vi "AT+TT.vi"(8 "错误输入（无错误）":errorcluster, 11 "站号":u16) -> (0 "错误输出":errorcluster)   [LabVIEW 2016, in "斯坦道原位多参数.lvlib"]
uses:
  <vilib>/Plasmionique/MB Master/MB_Master_Serial/MB_Master_Serial.lvclass/MB_Master_Serial.ctl
  <vilib>/Plasmionique/MB Master/MB_Master_Serial/Read VISA Resource.vi
  <vilib>/Plasmionique/MB Master/MB_VISA_Lock/MB_VISA_Lock.lvlib
  <vilib>/Plasmionique/MB Master/MB_Master_Serial/MB_Master_Serial.lvclass
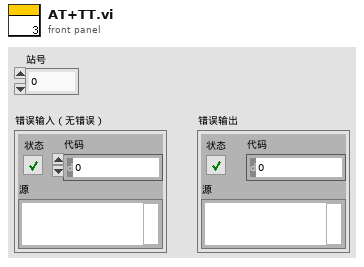
[diagram p1: front panel]
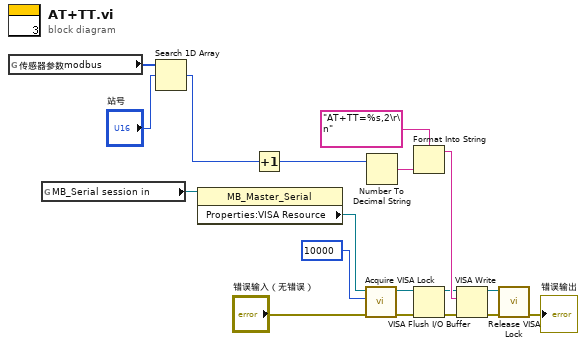
[diagram p0: block diagram]
diagram:
  n1 = global read "多参数断电保存全局变量.vi" "传感器参数modbus"() -> (w11:u16[])
  n2 = global read "多参数全局变量.vi" "MB_Serial session in"() -> (w9:refnum<class "MB_Master_Serial.lvclass">)
  n3 = Search 1D Array(1D array=w11, element="站号") -> (index of element=w17:i32)  [unwired: 1 in]
  n4 = property class="MB_Master_Serial"(reference=w9) -> ("Properties:VISA Resource"=w7:refnum<visa-resource-name>)  [unwired: 1 in, 2 out]
  n5 = Increment(x=w17) -> (x+1=w18:i32)
  n6 = call <vilib>:"Acquire VISA Lock.vi"("error in (no error)"="错误输入（无错误）", "timeout in ms (-1)"=10000, "VISA resource name"=w7) -> ("error out"=w5:errorcluster, "VISA resource name out"=w6:refnum<visa-resource-name>)  [unwired: 7 in]
  n7 = Number To Decimal String(number=w18) -> (decimal integer string=w12:string)  [unwired: 1 in]
  n8 = Format Into String(format string="AT+TT=%s,2\r\n" ("写入缓冲区"), w12) -> (resulting string=w13:string)  [unwired: 2 in, 1 out]
  n9 = VISA Flush I/O Buffer(VISA resource name=w6, error in (no error)=w5) -> (VISA resource name out=w4:refnum<visa-resource-name>, error out=w3:errorcluster)  [unwired: 1 in]
  n10 = VISA Write(VISA resource name=w4, write buffer=w13, error in (no error)=w3) -> (VISA resource name out=w2:refnum<visa-resource-name>, error out=w1:errorcluster)  [unwired: 1 out]
  n11 = call <vilib>:"Release VISA Lock.vi"("error in (no error)"=w1, "VISA resource name"=w2) -> ("error out"=→"错误输出":errorcluster)  [unwired: 8 in, 1 out]
